vi "patterns_square_shack_hartmann.vi"(1 "N":i32) -> (0 "Spots":T1[](array[typedef]) {"Amplitude Correction" step=0.1; "Line Trapping"."Phase Gradient" step=0.05; "Line Trapping"."Vector"."x" step=1e-06 format="%#_6p"; "Line Trapping"."Vector"."y" step=1e-06 format="%#_6p"; "Line Trapping"."Vector"."z" step=1e-06 format="%#_6p"; "NA Position"."r" step=1e-06; "NA Position"."y" step=1e-06; "NA Position"."x" step=1e-06; "Position"."z" step=1e-06; "Position"."y" step=1e-06; "Position"."x" step=1e-06; "Phase" step=0.7753; "Intensity" step=0.1})   [LabVIEW 2019]
uses:
  spot.ctl
  line_trapping.ctl
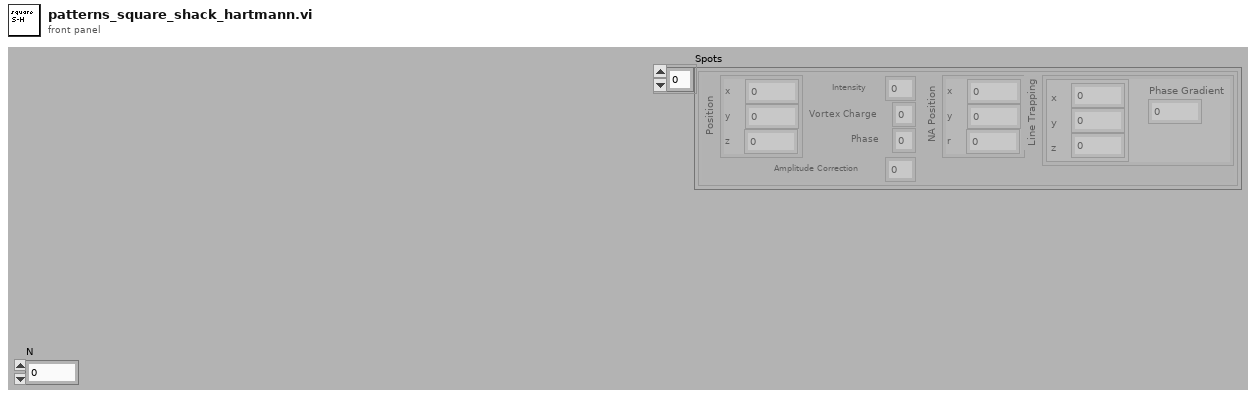
[diagram p1: front panel]
types:
  T1 = typedef "spot.ctl" = cluster{"Position":cluster{"x":dbl, "y":dbl, "z":dbl}, "Intensity":dbl, "Vortex Charge":i8, "Phase":dbl, "NA Position":cluster{"x":dbl, "y":dbl, "r":dbl}, "Line Trapping":T2, "Amplitude Correction":dbl}
  T2 = typedef "line_trapping.ctl" = cluster{"Vector":cluster{"x":dbl, "y":dbl, "z":dbl}, "Phase Gradient":dbl}
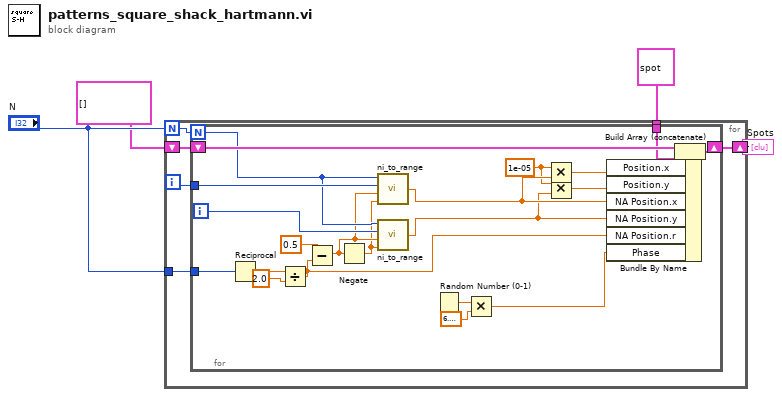
[diagram p0: block diagram]
diagram:
  n1 = for {
    N: "N" -> [w10]
    shift-right: [w7] -> w2
    shift-left: T1[] [] ("Spots 2") -> [w8]
    tunnel: T1 {"Position"={"x"=0.0, "y"=0.0, "z"=0.0}, "Intensity"=1.0, "Vortex Charge"=0, "Phase"=0.0, "NA Position"={"x"=0.0, "y"=0.0, "r"=1.0}, "Line Trapping"={"Vector"={"x"=0.0, "y"=0.0, "z"=0.0}, "Phase Gradient"=0.0}, "Amplitude Correction"=0.0} ("element") -> [w6]
    tunnel: "N" -> [w5]
    i -> [w9]
    n2 = for {
      N: w10 -> [w27]
      tunnel: w9 -> [w32]
      shift-right: [w31] -> w7
      shift-left: w8 -> [w30]
      tunnel: w6 -> [w28]
      tunnel: w5 -> [w11]
      i -> [w26]
      w23 = 1e-05 ("x")
      n3 = Reciprocal(x=w11) -> (1/x=w16:dbl)
      n4 = Divide(x=w16, y=2.0 ("x")) -> (x/y=w15:dbl)
      n5 = Subtract(x=0.5, y=w15) -> (x-y=w18:dbl)
      n6 = Negate(x=w18) -> (-x=w17:dbl)
      n7 = call "ni_to_range.vi"("end"=w17, "start"=w18, "i"=w32, "N"=w27) -> ("current value (runs from start to end in N steps)"=w24:dbl)
      n8 = call "ni_to_range.vi"("end"=w17, "start"=w18, "i"=w26, "N"=w27) -> ("current value (runs from start to end in N steps)"=w21:dbl)
      n9 = Random Number (0-1)() -> (number: 0 to 1=w14:dbl)
      n10 = Multiply(x=w14, y=6.283185307179586) -> (x*y=w12:dbl)
      n11 = Multiply(x=w23, y=w24) -> (x*y=w25:dbl)
      n12 = Multiply(x=w23, y=w21) -> (x*y=w22:dbl)
      n13 = Bundle By Name(cluster=w28, "Position.x"=w25, "Position.y"=w22, "NA Position.x"=w24, "NA Position.y"=w21, "NA Position.r"=w15, "Phase"=w12) -> (w29:T1)
      n14 = Build Array (concatenate)(w30, w29) -> (w31:T1[])
    }
  }
  "Spots" <- w2
